vi "TestStepProfile.vi"() -> ()   [LabVIEW 2016]
uses:
  <vilib>/Platform/TimedLoop/XDataNode/timing_clust.ctl
  <vilib>/Platform/TimedLoop/XDataNode/nitl_modes.ctl
  <vilib>/Platform/TimedLoop/XDataNode/wakeup.ctl
  <vilib>/Platform/TimedLoop/XDataNode/XDataNode.xnode
  <vilib>/Platform/TimedLoop/XDataNode/XDNodeRunTimeDep.lvlib
  Library/KevinLibraryAll/labview2011/kevLib2011.lvlib
panel:
  in  "Wait [10 ms]":i32=1000
  in  "Start Step":bool
  in  "Vac Step Size":sgl=50.0 min=0 max=100 step=1 format="%#_13g"
  in  "Increase":bool
  out "Waveform Chart":cluster{"number: 0 to 1":dbl, "upper limit":sgl}(graph)
  in  "stop":bool
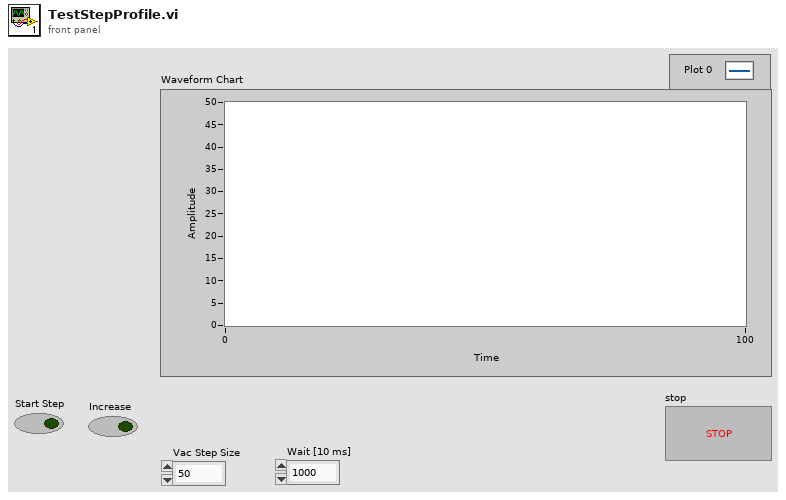
[diagram p1: front panel]
types:
  T1 = typedef "XDNodeRunTimeDep.lvlib/timing_clust.ctl" = cluster{"Expected End [f-1]":u64, "Actual End [f-1]":u64, "Finished Late? [f-1]":bool, "Expected End [i-1]":u64, "Actual End [i-1]":u64, "Finished Late? [i-1]":bool, "Expected Start [i]":u64, "Actual Start [i]":u64, "Expected Start [f]":u64, "Actual Start [f]":u64, "Source Name":string, "Structure Name":string, "Period":i64, "Deadline":i64, "Offset":i64, "Start":i64, "Priority":i32, "Timeout":i32, "Mode":T2, "Wakeup Reason":T3, "Error":errorcluster, "Source Type":string, "Secondary Source Type":string, "Global End Time":u64, "Global Start Time":u64, "Frame Duration":u64, "Iteration Duration":u64, "Assigned CPU":i32, "I/O Scan Engine Mode":u32}
  T2 = typedef "XDNodeRunTimeDep.lvlib/nitl_modes.ctl" = enum32{"No Change", "Process missed periods, maintain original phase", "Discard missed periods, maintain original phase", "Process missed periods, ignore original phase", "Discard missed periods, ignore original phase"}
  T3 = typedef "XDNodeRunTimeDep.lvlib/wakeup.ctl" = enum32{"Normal", "Aborted", "Asynchronous wakeup", "Timing source error", "Timed loop error", "Timeout"}
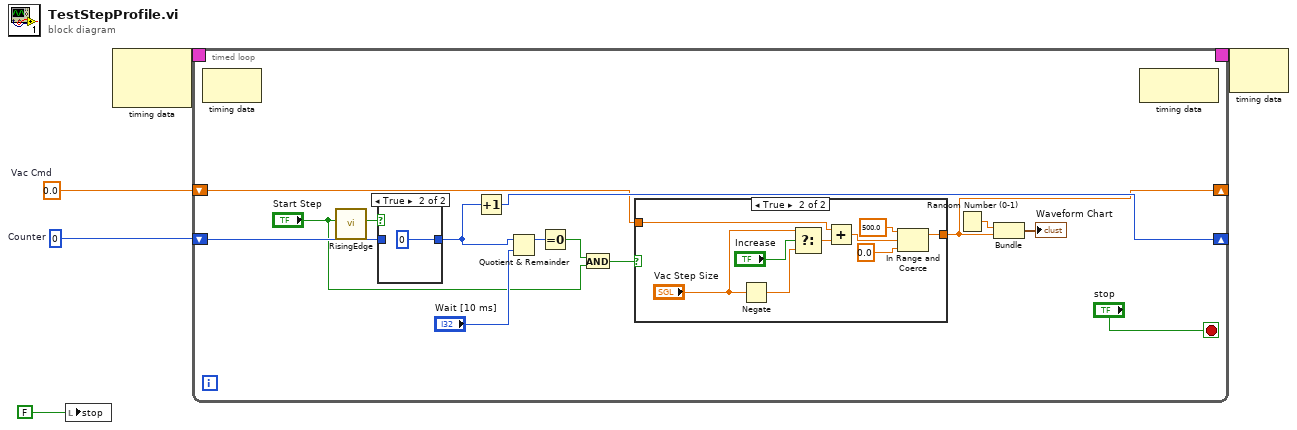
[diagram p0: block diagram]
diagram:
  w1 = 0  # Counter
  w2 = sgl 0.0  # Vac Cmd
  n1 = local write "stop"(FALSE ("stop")) -> ()
  n2 = node-c288() -> (w5:T1)  [unwired: 2 in]
  n3 = timed-loop {
    timing: w5 -> [_]
    timing-out: [_] -> w4
    shift-right: [w12] -> _
    shift-left: w1 -> [w13]
    shift-right: [w10] -> _
    shift-left: w2 -> [w11]
    stop <- "stop" stop-if-true
    n4 = node-c288() -> ()  [unwired: 1 in, 1 out]
    n5 = call "RisingEdge.vi"("Signal In"="Start Step") -> ("Rising Edge"=w18:bool)  [unwired: 10 in]
    n6 = case shown="True" w18 {
      tunnel: [w30 0] -> w6
      tunnel: w13 -> [w30 _]
      frame False {
      }
      frame True {
      }
    }
    n7 = Increment(x=w6) -> (x+1=w12:i32)
    n8 = Quotient & Remainder(x=w6, y="Wait [10 ms]") -> (x-y*floor(x/y)=w16:i32)  [unwired: 1 out]
    n9 = Equal To 0?(x=w16) -> (x = 0?=w9:bool)
    n10 = And(x=w9, y="Start Step") -> (x .and. y?=w8:bool)
    n11 = case shown="True" w8 {
      tunnel: [w20 w22] -> w10
      tunnel: w11 -> [w20 w21]
      frame False {
      }
      frame True {
        n12 = Negate(x="Vac Step Size") -> (-x=w29:sgl)
        n13 = Select(t="Vac Step Size", s="Increase", f=w29) -> (s? t:f=w27:sgl)
        n14 = Add(x=w21, y=w27) -> (x+y=w25:sgl)
        n15 = In Range and Coerce(upper limit=sgl 500.0, x=w25, lower limit=sgl 0.0) -> (coerced(x)=w22:sgl)  [unwired: 1 out]
      }
    }
    n16 = Random Number (0-1)() -> (number: 0 to 1=w14:dbl)
    n17 = Bundle("number: 0 to 1"=w14, "upper limit"=w10) -> (→"Waveform Chart":cluster{"number: 0 to 1":dbl, "upper limit":sgl})  [unwired: 1 in]
    n18 = node-c288() -> ()  [unwired: 1 in, 1 out]
  }
  n19 = node-c288(w4) -> ()  [unwired: 1 out]
